vi "Test_WriteMultiple_RetrieveAll.vi"(8 "error in (no error)":errorcluster, 11 "TestCase in":refnum<class "TestCurrentValueTable.lvclass">) -> (0 "error out":errorcluster, 3 "TestCase out":refnum<class "TestCurrentValueTable.lvclass">)   [LabVIEW 2015, in "CurrentValueTable.lvlib" / "TestCurrentValueTable.lvclass"]
uses:
  TestCurrentValueTable.lvclass
  <vilib>/addons/_JKI Toolkits/VI Tester/TestCase.llb/TestCase.lvclass
  CurrentValueTable.lvclass
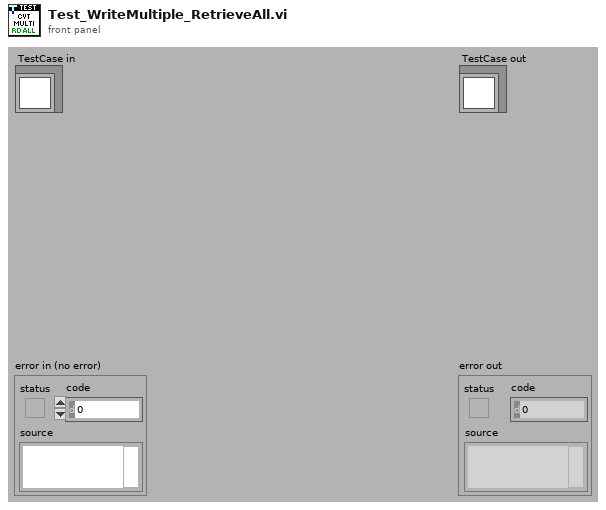
[diagram p1: front panel]
types:
  T1 = typedef "CurrentValueTable.lvlib/CurrentValueTable.lvclass/CurrentValueTable Reference.ctl" = refnum<data-value>
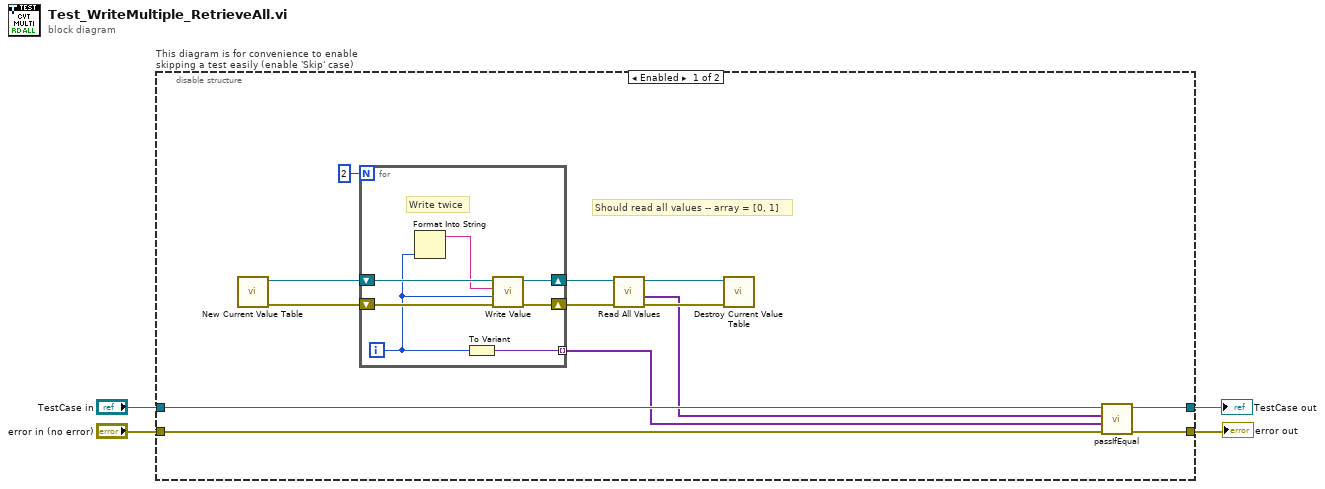
[diagram p0: block diagram]
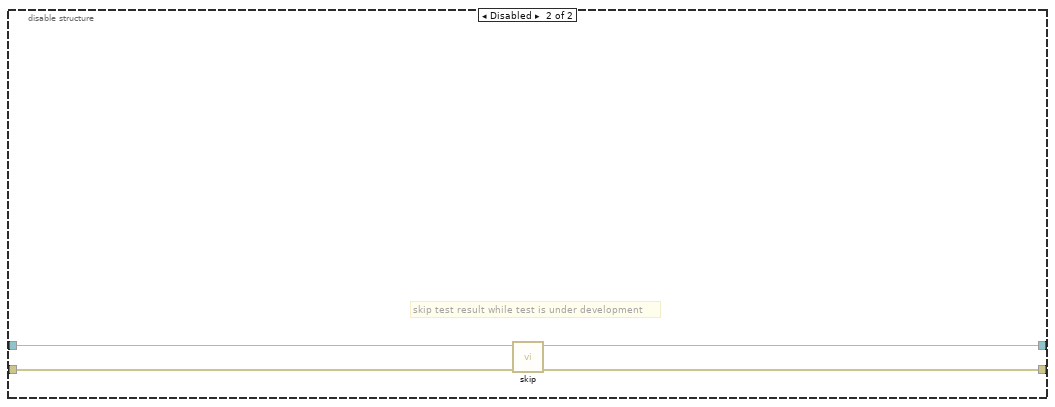
[diagram p2: hidden frame]
diagram:
  n1 = disable-structure "This diagram is for convenience to enable skipping a test easily (enable 'Skip' case)" shown="Enabled" {
    disable-tunnel: "TestCase in" -> [w17 w28]
    disable-tunnel: [w16 w26] -> w1
    disable-tunnel: [w15 w27] -> w3
    disable-tunnel: "error in (no error)" -> [w14 w25]
    frame Enabled {
      # "Should read all values -- array = [0, 1]"
      n2 = call "New Current Value Table.vi"() -> ("error out"=w11:errorcluster, "Current Value Table"=w13:T1)  [unwired: 10 in]
      n3 = for {
        N: 2 -> [_]
        shift-right: [w23] -> w12
        shift-left: w13 -> [w24]
        shift-right: [w21] -> w8
        shift-left: w11 -> [w22]
        tunnel: [w18] -> w5 mode=indexing
        i -> [w20]
        # "Write twice"
        n4 = Format Into String(w20) -> (resulting string=w19:string)  [unwired: 3 in, 1 out]
        n5 = To Variant(anything=w20) -> (Variant=w18:variant)
        n6 = call "Write Value.vi"("error in (no error)"=w22, "Value"=w20, "Data Name (Use Value Name)"=w19, "Current Value Table"=w24) -> ("error out"=w21:errorcluster, "Current Value Table"=w23:T1)  [unwired: 6 in]
      }
      n7 = call "Read All Values.vi"("error in (no error)"=w8, "Current Value Table"=w12) -> ("error out"=w7:errorcluster, "Values"=w6:variant[], "Current Value Table"=w9:T1)  [unwired: 6 in, 1 out]
      n8 = call "Destroy Current Value Table.vi"("error in (no error)"=w7, "Current Value Table"=w9) -> ()  [unwired: 9 in, 1 out]
      n9 = call-dynamic "passIfEqual.vi"("error in (no error)"=w14, "y"=w5, "x"=w6, "TestCase in"=w17) -> ("error out"=w15:errorcluster, "TestCase out"=w16:refnum<class "TestCurrentValueTable.lvclass">)  [unwired: 6 in]
    }
    frame Disabled {
      # "skip test result while test is under development"
      n10 = call <vilib>:"skip.vi"("error in (no error)"=w25, "TestCase in"=w28) -> ("error out"=w27:errorcluster, "TestCase out"=w26:refnum<class "TestCurrentValueTable.lvclass">)  [unwired: 8 in]
    }
  }
  "error out" <- w3
  "TestCase out" <- w1
